vi "Popup Message.vi"(8 "error in (no error)":errorcluster, 9 "Duration (s) (6)":u32=6, 10 "Message Type (INFO)":enum16{"INFO", "WARNING", "ERROR"}(ring), 11 "Message":string) -> (0 "error out":errorcluster)   [LabVIEW 2011, in "COSYLib.lvlib"]
uses:
  COSYLib.lvlib
  Popup Message CORE.vi
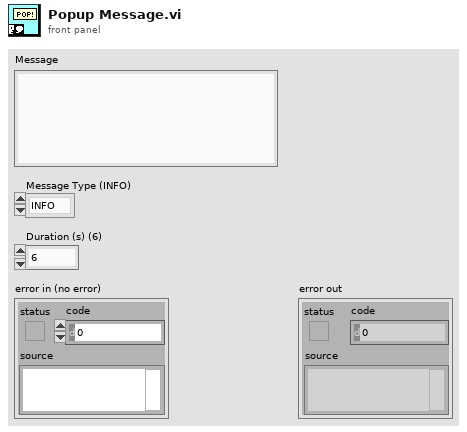
[diagram p1: front panel]
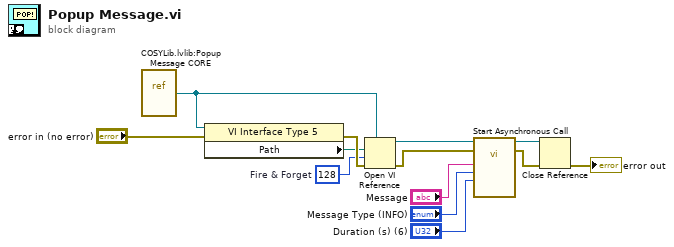
[diagram p0: block diagram]
diagram:
  w9 = 128  # Fire & Forget
  n1 = vi-ref "COSYLib.lvlib:Popup Message CORE.vi"() -> (w10:refnum<vi>)
  n2 = property class="VI Interface Type 5"(reference=w10, error in="error in (no error)") -> (error out=w12:errorcluster, "Path"=w11:path)  [unwired: 1 out]
  n3 = Open VI Reference(type specifier VI Refnum (for type only)=w10, vi path=w11, options=w9, error in (no error)=w12) -> (vi reference=w8:refnum<vi>, error out=w6:errorcluster)  [unwired: 2 in]
  n4 = call-by-ref "Start Asynchronous Call"(reference=w8, error in=w6, "Duration (s)"="Duration (s) (6)", "Message Type"="Message Type (INFO)", "Message"="Message") -> (reference out=w7:refnum<vi>, error out=w2:errorcluster)  [unwired: 9 in]
  n5 = Close Reference(reference=w7, error in (no error)=w2) -> (error out=→"error out":errorcluster)
